vi "Device configured.vi"(2 "error in (no error)":errorcluster, 3 "handle":u32) -> (0 "error out":errorcluster, 1 "ready":bool)   [LabVIEW 2013]
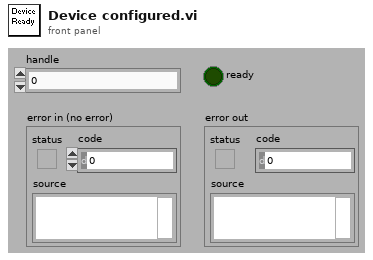
[diagram p1: front panel]
types:
  T1 = cluster{"Pin 1":bool, "Pin 2":bool, "Pin 3":bool, "Pin 4":bool, "Pin 5":bool, "Pin 6":bool, "Pin 7":bool, "Pin 8":bool}
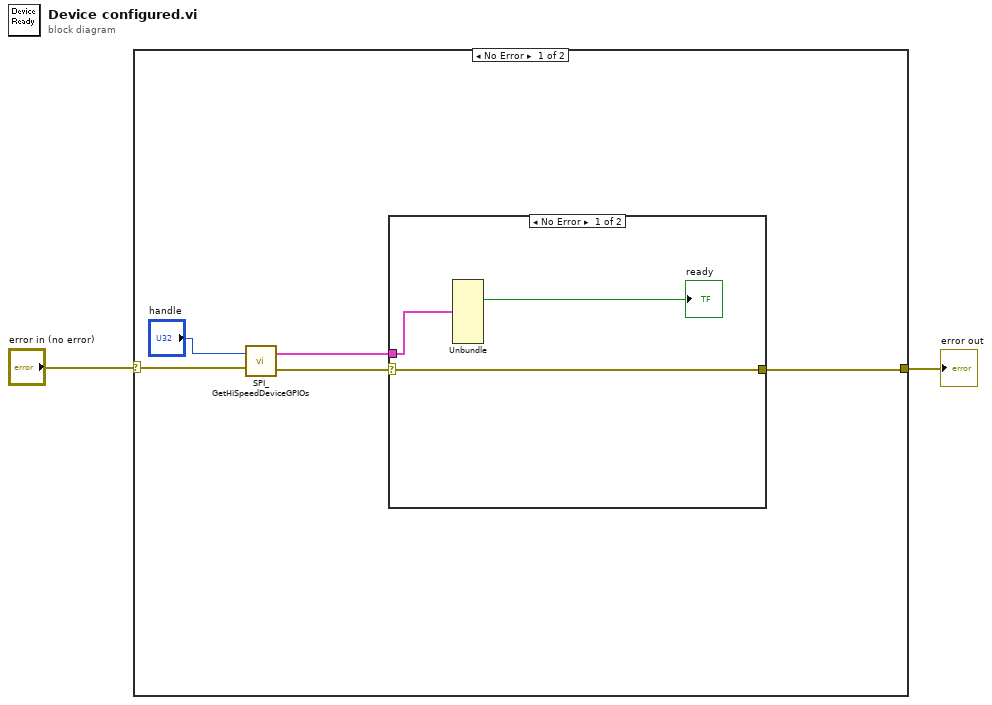
[diagram p0: block diagram]
diagram:
  n1 = case shown="No Error" "error in (no error)" {
    selector: "error in (no error)" -> [w7 w12]
    tunnel: [w3 w12] -> w1
    frame No Error {
      n2 = call "SPI_GetHiSpeedDeviceGPIOs.vi"("error in (no error)"=w7, "handle"="handle") -> ("error out"=w5:errorcluster, "high pins input data"=w4:T1)
      n3 = case shown="No Error" w5 {
        selector: w5 -> [w10 w11]
        tunnel: w4 -> [w9 _]
        tunnel: [w10 w11] -> w3
        frame No Error {
          n4 = Unbundle(w9) -> ("Pin 3"=→"ready":bool)  [unwired: 7 out]
        }
        frame Error {
        }
      }
    }
    frame Error {
    }
  }
  "error out" <- w1
